vi "Run.vi"(8 "error in (no error)":errorcluster, 9 "s on last turn":dbl, 10 "Maze (0: Empty, -1: Enemy. >0: Teammate":i32[][](array[numeric]), 11 "Attack in":refnum<class "Attack.lvclass">) -> (0 "error out":errorcluster, 1 "Direction":T1, 2 "Action":T2, 3 "Attack out":refnum<class "Attack.lvclass">, 4 "Replicated":refnum<class "Runner.lvclass">)   [LabVIEW 2014, in "Attack.lvclass"]
uses:
  Attack.lvclass
  Action Enum.ctl
  Direction Enum.ctl
  Runner.lvclass
  Attack.lvclass/Attack.ctl
  Spawn/Spawn.lvclass
  SquareBattle.lvclass
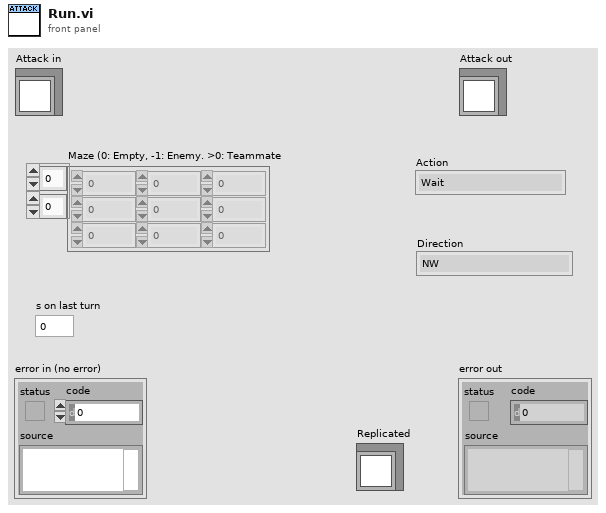
[diagram p1: front panel]
types:
  T1 = typedef "SquareBattle.lvclass/Direction Enum.ctl" = enum16{"NW", "N", "NE", "E", "SE", "S", "SW", "W"}
  T2 = typedef "SquareBattle.lvclass/Action Enum.ctl" = enum16{"Wait", "Move", "Attack", "Replicate"}
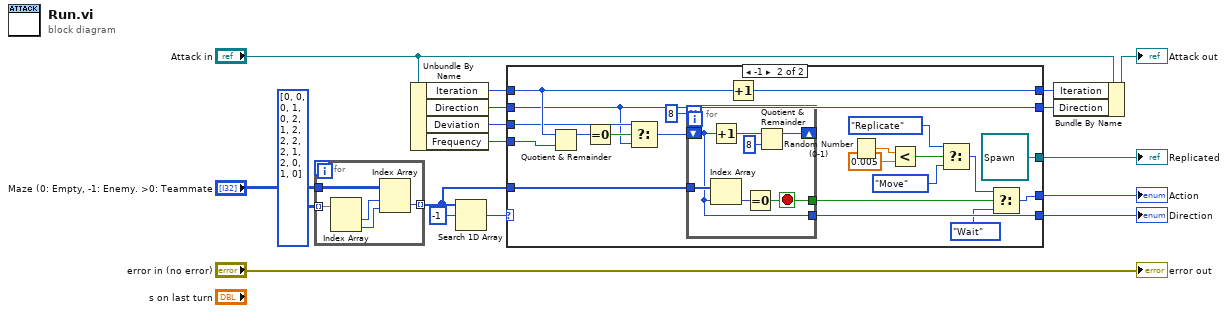
[diagram p0: block diagram]
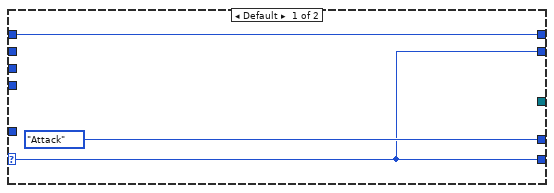
[diagram p2: hidden frame]
diagram:
  n1 = for {
    tunnel: "Maze (0: Empty, -1: Enemy. >0: Teammate" -> [w22]
    tunnel: i32[][] [[0, 0], [0, 1], [0, 2], [1, 2], [2, 2], [2, 1], [2, 0], [1, 0]] -> [w21] mode=indexing
    tunnel: [w18] -> w3 mode=indexing
    n2 = Index Array(array=w21) -> (element #1=w20:i32, element #2=w19:i32)  [unwired: 2 in]
    n3 = Index Array(array=w22, index (row)=w20, index (col)=w19) -> (element=w18:i32)
  }
  n4 = Unbundle By Name("Attack in") -> ("Iteration"=w10:i32, "Direction"=w6:T1, "Deviation"=w5:T1, "Frequency"=w4:i32)
  n5 = Search 1D Array(1D array=w3, element=-1) -> (index of element=w13:i32)  [unwired: 1 in]
  n6 = case shown="-1" w13 {
    selector: w13 -> [w23 _]
    tunnel: [w23 w37] -> w12
    tunnel: [Action_Enum."Attack" ("Action") w31] -> w11
    tunnel: w10 -> [w24 w45]
    tunnel: [w24 w46] -> w9
    tunnel: w6 -> [_ w34]
    tunnel: w5 -> [_ w41]
    tunnel: w4 -> [_ w44]
    tunnel: w3 -> [_ w40]
    tunnel: [w23 w34] -> w2
    tunnel: [_ refnum<class "Spawn.lvclass"> refnum ("Spawn.lvclass")] -> w1
    frame Default {
    }
    frame -1 {
      n7 = Quotient & Remainder(x=w45, y=w44) -> (x-y*floor(x/y)=w43:i32)  [unwired: 1 out]
      n8 = Equal To 0?(x=w43) -> (x = 0?=w42:bool)
      n9 = Select(t=w41, s=w42, f=w34) -> (s? t:f=w38:T1)
      n10 = for {
        N: 8 -> [_]
        tunnel: w40 -> [w53]
        shift-right: [w49] -> _
        shift-left: w38 -> [w48]
        tunnel: [w48] -> w37
        tunnel: [w47] -> w36
        stop <- w47 stop-if-true
        n11 = Increment(x=w48) -> (x+1=w51:i32)
        n12 = Index Array(array=w53, index=w48) -> (element=w52:i32)
        n13 = Equal To 0?(x=w52) -> (x = 0?=w47:bool)
        n14 = Quotient & Remainder(x=w51, y=8) -> (x-y*floor(x/y)=w49:i32)  [unwired: 1 out]
      }
      n15 = Increment(x=w45) -> (x+1=w46:i32)
      n16 = Random Number (0-1)() -> (number: 0 to 1=w33:dbl)
      n17 = Less?(x=w33, y=0.005) -> (x < y?=w30:bool)
      n18 = Select(t=Action_Enum."Replicate" ("Action"), s=w30, f=Action_Enum."Move" ("Action")) -> (s? t:f=w28:T2)
      n19 = Select(t=w28, s=w36, f=Action_Enum."Wait" ("Action")) -> (s? t:f=w31:T2)
    }
  }
  "Action" <- w11
  "Direction" <- w12
  "Replicated" <- w1
  n20 = Bundle By Name(cluster="Attack in", "Iteration"=w9, "Direction"=w2) -> (→"Attack out":refnum<class "Attack.lvclass">)
  "error out" <- "error in (no error)"
